vi "geraChecksum.vi"(7 "Soma":u16) -> (8 "checksum":u8)   [LabVIEW 2018]
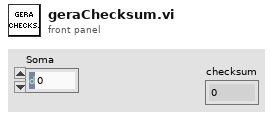
[diagram p1: front panel]
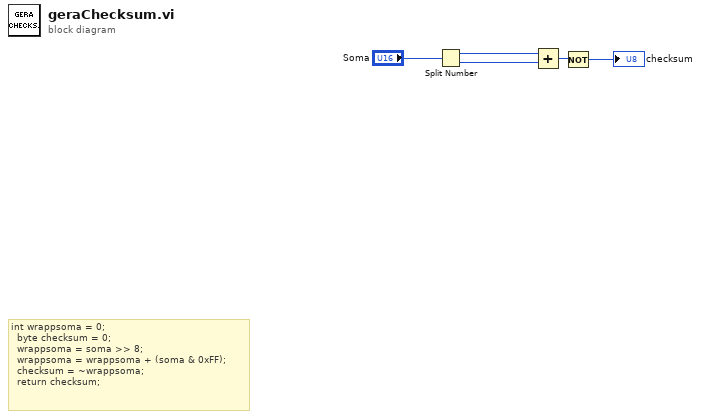
[diagram p0: block diagram]
diagram:
  # "int wrappsoma = 0;\n  byte checksum = 0;\n  wrappsoma = soma >> 8;\n  wrappsoma = wrappsoma + (soma & 0xFF);\n  checksum = ~wrappsoma;\n  return checksum;"
  n1 = Split Number(x="Soma") -> (hi(x)=w2:u8, lo(x)=w1:u8)
  n2 = Add(x=w2, y=w1) -> (x+y=w5:u8)
  n3 = Not(x=w5) -> (.not. x?=→"checksum":u8)
